vi "DAQ.vi"(0 "Handle In":i32, 1 "TC1 Type":u16(ring)=7 items=["B", "E", "J", "K", "N", "R", "S", "T"], 2 "TC1 +Channel":u16, 3 "TC1 -Channel":u16=1, 4 "TC2 Type":u16(ring)=3 items=["B", "E", "J", "K", "N", "R", "S", "T"], 5 "TC2 +Channel":u16=2, 6 "TC2 -Channel":u16=3, 7 "error in":errorcluster, 8 "LP1 Pin":u16=10, 9 "k [N/m]":dbl=2000.0, 12 "PT1 Pin":u16=8, 13 "PT2 Pin":u16=6, 14 "PT3 Pin":u16=4, 15 "Solenoid Supply Pin":u16=5, 16 "LabJack Supply Pin":u16=7, 17 "Relay Supply Pin":u16=9, 18 "Deadman Switch Pin":u16(ring) items=["FIO0", "FIO1", "FIO2", "FIO3", "FIO4", "FIO5", "FIO6", "FIO7", "EIO0", "EIO1", "EIO2", "EIO3", "EIO4", "EIO5", "EIO6", "EIO7", "CIO0", "CIO1", "CIO2", "CIO3", "MIO0", "MIO1", "MIO2"]) -> (25 "Sensor Values":dbl[](array[numeric]), 26 "Deadman Switch":bool, 27 "error out":errorcluster[](array[cluster]))   [LabVIEW 2021]
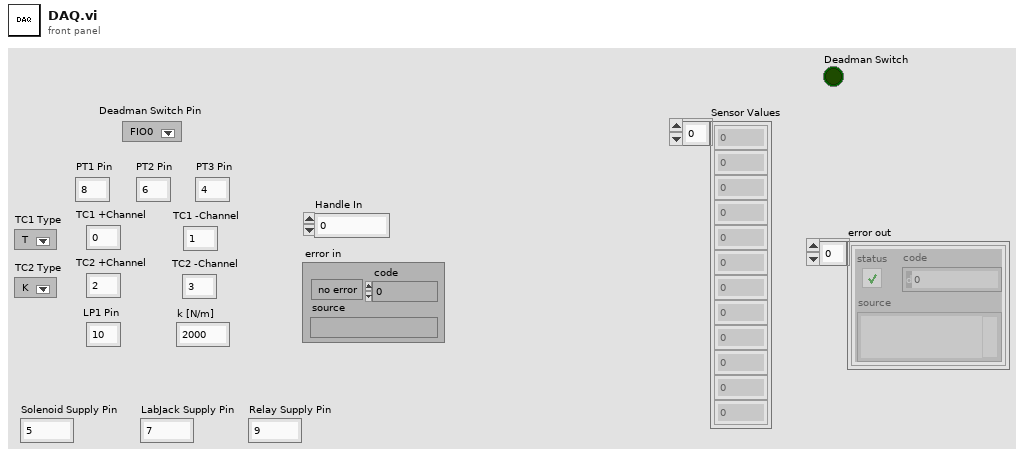
[diagram p1: front panel]
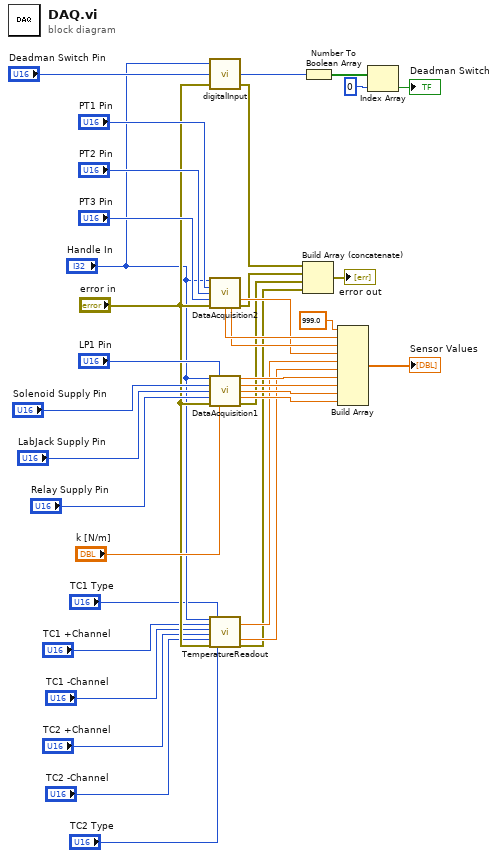
[diagram p0: block diagram]
diagram:
  n1 = call "digitalInput.vi"("error in"="error in", "Channel"="Deadman Switch Pin", "Handle In"="Handle In") -> ("error out"=w14:errorcluster, "State"=w28:i32)  [unwired: 1 out]
  n2 = call "DataAcquisition2.vi"("Handle In"="Handle In", "PT1 Pin"="PT1 Pin", "PT2 Pin"="PT2 Pin", "PT3 Pin"="PT3 Pin", "error in"="error in") -> ("PT3 Pressure Reading"=w21:dbl, "PT1 Pressure Reading"=w23:dbl, "PT2 Pressure Reading"=w22:dbl, "error out"=w2:errorcluster[])  [unwired: 2 in, 5 out]
  n3 = call "DataAcquisition1.vi"("Handle In"="Handle In", "LP1 Pin"="LP1 Pin", "Solenoid Supply Pin"="Solenoid Supply Pin", "LabJack Supply Pin"="LabJack Supply Pin", "Relay Supply Pin"="Relay Supply Pin", "error in"="error in", "k"="k [N/m]") -> ("Thrust Reading [Newton]"=w20:dbl, "Solenoid Supply Voltage"=w19:dbl, "LabJack Supply Voltage"=w18:dbl, "Relay Supply Voltage"=w17:dbl, "error out"=w1:errorcluster[])  [unwired: 2 in, 2 out]
  n4 = call "TemperatureReadout.vi"("Handle In"="Handle In", "TC1 +Channel"="TC1 +Channel", "TC1 -Channel"="TC1 -Channel", "TC2 +Channel"="TC2 +Channel", "TC2 -Channel"="TC2 -Channel", "error in"="error in", "TC1 Type"="TC1 Type", "TC2 Type"="TC2 Type") -> ("TC1 Temperature (Kelvin)"=w12:dbl, "TC2 Temperature (Kelvin)"=w11:dbl, "error out"=w3:errorcluster[])  [unwired: 3 in, 6 out]
  n5 = Build Array (concatenate)(w14, w2, w1, w3) -> (→"error out":errorcluster[])
  n6 = Number To Boolean Array(number=w28) -> (Boolean array=w27:bool[])
  n7 = Build Array(999.0 ("element"), w23, w22, w21, w12, w11, w20, w19, w18, w17) -> (→"Sensor Values":dbl[])
  n8 = Index Array(array=w27, index=0) -> (element=→"Deadman Switch":bool)
